vi "Data Server Demo.vi"(8 "error in":errorcluster) -> (0 "error out":errorcluster)   [LabVIEW 2012]
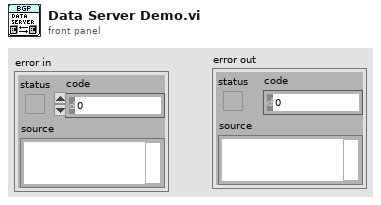
[diagram p1: front panel]
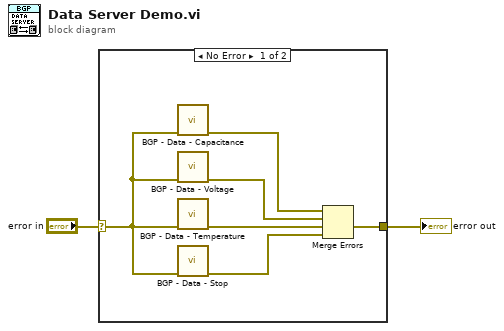
[diagram p0: block diagram]
diagram:
  n1 = case shown="No Error" "error in" {
    selector: "error in" -> [w3 w9]
    tunnel: [w6 w9] -> w2
    frame No Error {
      n2 = call "BGP - Data - Capacitance.vi"("error in"=w3) -> ("error out"=w4:errorcluster)  [unwired: 10 in]
      n3 = call "BGP - Data - Voltage.vi"("error in"=w3) -> ("error out"=w5:errorcluster)  [unwired: 10 in]
      n4 = call "BGP - Data - Temperature.vi"("error in"=w3) -> ("error out"=w8:errorcluster)  [unwired: 10 in]
      n5 = call "BGP - Data - Stop.vi"("error in (no error)"=w3) -> ("error out"=w7:errorcluster)  [unwired: 10 in]
      n6 = Merge Errors(w4, w5, w8, w7) -> (w6:errorcluster)
    }
    frame Error {
    }
  }
  "error out" <- w2
